vi "PIV_Interpolate.vi"(8 "error in (no error)":errorcluster, 9 "post-processing":T2={"mask threshold"=1.02, "method"="", "max iteration"=0, "kernal size"=0}, 11 "raw":T1) -> (0 "error out":errorcluster={"status"=TRUE, "code"=1671, "source"="Python Node in PIV_Pixel.vi->LabVIEW_GUI.vi<APPEND>\n\nModule Path: /Users/crogers/Desktop/PIV/LabVIEW/subs/code.py\nFunction Name: piv\nPython returned the following error: <class 'OSError'>\nImageIO does not generally support reading folders. Limited support may be available via specific plugins. Specify the plugin explicitly using the `plugin` kwarg, e.g. `plugin='DICOM'`\n\n\n Call Stack information:\n['Traceback (most recent call last):\n', '  File \"/Users/crogers/Desktop/PIV/LabVIEW/subs/code.py\", line 8, in piv\n    frame_a = tools.imread(path_t)\n', '  File \"/Users/crogers/Library/Python/3.10/lib/python/site-packages/openpiv/tools.py\", line 337, in imread\n    im = _imread(filename)\n', '  File \"/Users/crogers/Library/Python/3.10/lib/python/site-packages/imageio/v3.py\", line 53, in imread\n    with imopen(uri, \"r\", **plugin_kwargs) as img_file:\n', '  File \"/Users/crogers/Library/Python/3.10/lib/python/site-packages/imageio/core/imopen.py\", line 223, in imopen\n    raise err_type(err_msg)\n', \"OSError: ImageIO does not generally support reading folders. Limited support may be available via specific plugins. Specify the plugin explicitly using the `plugin` kwarg, e.g. `plugin='DICOM'`\n\"]"}, 3 "interpolated":T1)   [LabVIEW 2025]
uses:
  PIV_postParameters.ctl
  PIV_velocities.ctl
panel:
  out "mask":i16[][](graph)
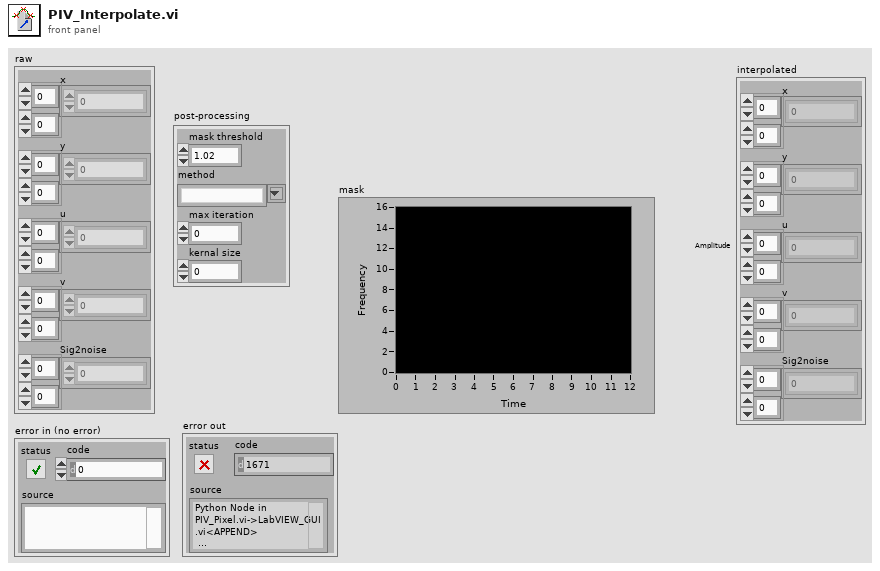
[diagram p1: front panel]
types:
  T1 = typedef "PIV_velocities.ctl" = cluster{"x":dbl[][], "y":dbl[][], "u":dbl[][], "v":dbl[][], "Sig2noise":dbl[][]}
  T2 = typedef "PIV_postParameters.ctl" = cluster{"mask threshold":dbl, "method":string, "max iteration":u8, "kernal size":u8}
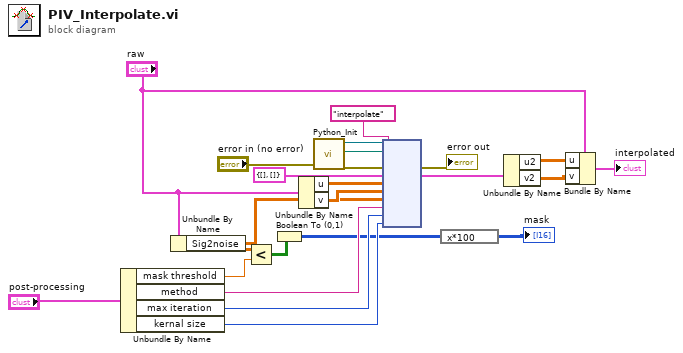
[diagram p0: block diagram]
diagram:
  n1 = Unbundle By Name("post-processing") -> ("mask threshold"=w14:dbl, "method"=w13:string, "max iteration"=w12:u8, "kernal size"=w11:u8)
  n2 = Unbundle By Name("raw") -> ("Sig2noise"=w4:dbl[][])
  n3 = Less?(x=w4, y=w14) -> (x < y?=w15:bool[][])
  n4 = Boolean To (0,1)(Boolean=w15) -> (0, 1=w6:i16[][])
  n5 = Unbundle By Name("raw") -> ("u"=w3:dbl[][], "v"=w16:dbl[][])
  n6 = call "Python_Init.vi"("error in (no error)"="error in (no error)") -> ("Refnum out"=w22:refnum<k35>, "code"=w19:path, "error out"=w23:errorcluster)  [unwired: 3 in]
  n7 = node(w22, w19, "interpolate" ("function name"), w23, cluster{"u2":dbl[][], "v2":dbl[][]} {"u2"=[], "v2"=[]}, w3, w16, w4, w13, w12, w11) -> (→"error out":errorcluster, w1:cluster{"u2":dbl[][], "v2":dbl[][]})  [unwired: 6 in, 3 out]
  n8 = expression code="x*100"(w6) -> (→"mask":i16[][])
  n9 = Unbundle By Name(w1) -> ("u2"=w9:dbl[][], "v2"=w8:dbl[][])
  n10 = Bundle By Name(cluster="raw", "u"=w9, "v"=w8) -> (→"interpolated":T1)
